vi "Substitute Panel VI.vi"(7 "VI Reference":refnum<vi>, 10 "SubPanel Reference":refnum<vi>) -> (0 "error out":errorcluster)   [LabVIEW 2016, in "Assert Display.lvlib" / "Base UI Component.lvlib" / "Base UI Component.lvclass"]
uses:
  Base UI Component.lvclass
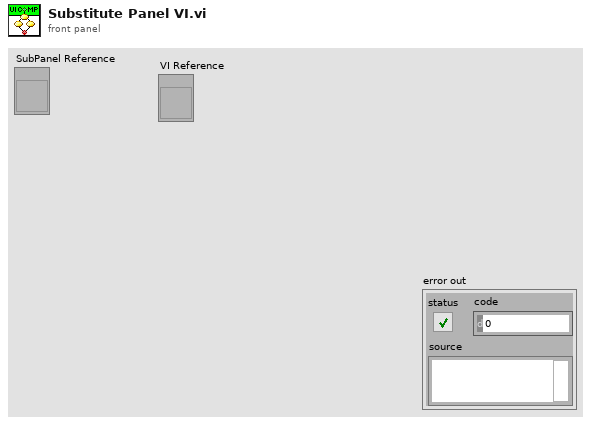
[diagram p1: front panel]
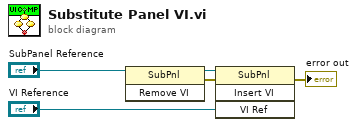
[diagram p0: block diagram]
diagram:
  n1 = invoke class="SubPnl" method="Remove VI"(reference="SubPanel Reference") -> (reference out=w5:refnum<vi>, error out=w4:errorcluster)  [unwired: 2 in, 1 out]
  n2 = invoke class="SubPnl" method="Insert VI"(reference=w5, error in=w4, "VI Ref"="VI Reference") -> (error out=→"error out":errorcluster)  [unwired: 1 in, 3 out]
